vi "servo-arm.vi"   [LabVIEW 2016, in "Moving Motor.lvrbt"]
uses:
  Moving Motor.lvrbt
  <vilib>/NXT/Hardware/Plugins/Tetrix 180 deg Servo/Tetrix180ServoAddress.ctl
  <vilib>/NXT/NXTIO Xnodes/NXTIONodeSubVIs/TETRIX IO Move Servos.vi
  <vilib>/NXT/Dual Mode Library/Waits/Wait_Num(msec).vi
  <vilib>/NXT/NXTIO Xnodes/AddressXNode/NXTIOAddress.xnode
  <vilib>/NXT/Subs/LVHSConnector.ctl
  <vilib>/NXT/NXTIO Xnodes/NXTIOXNode/NXTIO.xnode
  <vilib>/NXT/LegoClasses/BrickReference/BrickReference.lvclass
types:
  T1 = typedef "Tetrix180ServoAddress.ctl" = i32
  T2 = cluster{"Tetrix180Servo":T1, "Tetrix180Servo":T1}
  T3 = typedef "LVHSConnector.ctl" = refnum<class "BrickReference.lvclass">
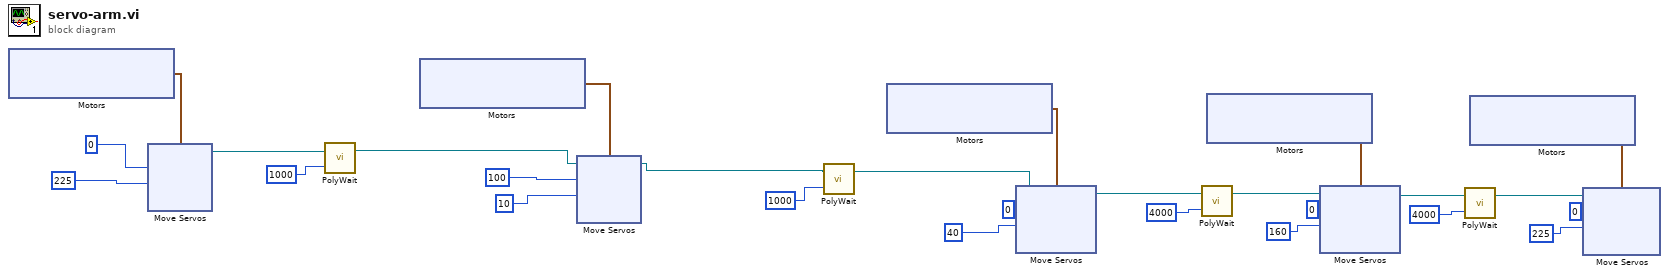
[diagram p0: block diagram]
diagram:
  n1 = xnode "Motors"() -> ("Motor"=w23:T2)
  n2 = xnode "Move Servos"("Position 2"=u8 225, "Position 1"=u8 0, "Motors"=w23) -> ("NXT/EV3"=w18:T3)  [unwired: 1 in]
  n3 = call-poly <vilib>:"PolyWait.vi"("Time (100 msec)"=u32 1000, "NXT/EV3"=w18) -> ("NXT/EV3"=w19:T3)  [unwired: 2 in]
  n4 = xnode "Motors"() -> ("Motor"=w26:T2)
  n5 = xnode "Move Servos"("Position 2"=u8 10, "Position 1"=u8 100, "Motors"=w26, "NXT/EV3"=w19) -> ("NXT/EV3"=w17:T3)
  n6 = call-poly <vilib>:"PolyWait.vi"("Time (100 msec)"=u32 1000, "NXT/EV3"=w17) -> ("NXT/EV3"=w15:T3)  [unwired: 2 in]
  n7 = xnode "Motors"() -> ("Motor"=w16:T2)
  n8 = xnode "Move Servos"("Position 2"=u8 40, "Position 1"=u8 0, "Motors"=w16, "NXT/EV3"=w15) -> ("NXT/EV3"=w11:T3)
  n9 = call-poly <vilib>:"PolyWait.vi"("Time (100 msec)"=u32 4000, "NXT/EV3"=w11) -> ("NXT/EV3"=w7:T3)  [unwired: 2 in]
  n10 = xnode "Motors"() -> ("Motor"=w12:T2)
  n11 = xnode "Move Servos"("Position 2"=u8 160 ("Position 1"), "Position 1"=u8 0, "Motors"=w12, "NXT/EV3"=w7) -> ("NXT/EV3"=w1:T3)
  n12 = call-poly <vilib>:"PolyWait.vi"("Time (100 msec)"=u32 4000, "NXT/EV3"=w1) -> ("NXT/EV3"=w2:T3)  [unwired: 2 in]
  n13 = xnode "Motors"() -> ("Motor"=w6:T2)
  n14 = xnode "Move Servos"("Position 2"=u8 225 ("Position 1"), "Position 1"=u8 0, "Motors"=w6, "NXT/EV3"=w2) -> ()  [unwired: 1 out]
